vi "Sekvenca (SubVI).vi"(11 "Ulaz":dbl) -> (3 "Cluster 41":cluster{"Path":path, "Array":dbl[]})   [LabVIEW 2012]
panel:
  in  "Cluster 40":cluster{"Path":path, "Array":dbl[]}={"Path"=path "40.wav", "Array"=[1.0, 2.0]}
  in  "Cluster 39":cluster{"Path":path, "Array":dbl[]}={"Path"=path "39.wav", "Array"=[1.0, 2.0]}
  in  "Cluster 38":cluster{"Path":path, "Array":dbl[]}={"Path"=path "38.wav", "Array"=[1.0, 1.0, 2.0, 1.0]}
  in  "Cluster 37":cluster{"Path":path, "Array":dbl[]}={"Path"=path "37.wav", "Array"=[1.0, 1.0, 2.0, 1.0]}
  in  "Cluster 36":cluster{"Path":path, "Array":dbl[]}={"Path"=path "36.wav", "Array"=[2.0, 1.0]}
  in  "Cluster 35":cluster{"Path":path, "Array":dbl[]}={"Path"=path "35.wav", "Array"=[2.0, 1.0]}
  in  "Cluster 34":cluster{"Path":path, "Array":dbl[]}={"Path"=path "34.wav", "Array"=[4.0, 1.0]}
  in  "Cluster 33":cluster{"Path":path, "Array":dbl[]}={"Path"=path "33.wav", "Array"=[4.0]}
  in  "Cluster 32":cluster{"Path":path, "Array":dbl[]}={"Path"=path "32.wav", "Array"=[1.0]}
  in  "Cluster 31":cluster{"Path":path, "Array":dbl[]}={"Path"=path "31.wav", "Array"=[1.0]}
  in  "Cluster 30":cluster{"Path":path, "Array":dbl[]}={"Path"=path "30.wav", "Array"=[1.0]}
  in  "Cluster 29":cluster{"Path":path, "Array":dbl[]}={"Path"=path "29.wav", "Array"=[1.0]}
  in  "Cluster 28":cluster{"Path":path, "Array":dbl[]}={"Path"=path "28.wav", "Array"=[1.0, 1.0]}
  in  "Cluster 27":cluster{"Path":path, "Array":dbl[]}={"Path"=path "27.wav", "Array"=[1.0, 1.0]}
  in  "Cluster 26":cluster{"Path":path, "Array":dbl[]}={"Path"=path "26.wav", "Array"=[1.0, 1.0, 2.0]}
  in  "Cluster 25":cluster{"Path":path, "Array":dbl[]}={"Path"=path "25.wav", "Array"=[1.0, 1.0, 2.0]}
  in  "Cluster 24":cluster{"Path":path, "Array":dbl[]}={"Path"=path "24.wav", "Array"=[1.0, 1.0]}
  in  "Cluster 23":cluster{"Path":path, "Array":dbl[]}={"Path"=path "23.wav", "Array"=[1.0, 1.0]}
  in  "Cluster 22":cluster{"Path":path, "Array":dbl[]}={"Path"=path "22.wav", "Array"=[2.0, 3.0, 2.0]}
  in  "Cluster 21":cluster{"Path":path, "Array":dbl[]}={"Path"=path "21.wav", "Array"=[1.0, 1.0, 2.0]}
  in  "Cluster 20":cluster{"Path":path, "Array":dbl[]}={"Path"=path "20.wav", "Array"=[1.0, 1.0, 2.0, 1.0]}
  in  "Cluster 19":cluster{"Path":path, "Array":dbl[]}={"Path"=path "19.wav", "Array"=[1.0, 2.0, 1.0, 1.0]}
  in  "Cluster 18":cluster{"Path":path, "Array":dbl[]}={"Path"=path "18.wav", "Array"=[1.0, 2.0, 1.0]}
  in  "Cluster 17":cluster{"Path":path, "Array":dbl[]}={"Path"=path "17.wav", "Array"=[1.0, 2.0]}
  in  "Cluster 16":cluster{"Path":path, "Array":dbl[]}={"Path"=path "16.wav", "Array"=[1.0, 1.0, 1.0]}
  in  "Cluster 15":cluster{"Path":path, "Array":dbl[]}={"Path"=path "15.wav", "Array"=[1.0, 1.0]}
  in  "Cluster 14":cluster{"Path":path, "Array":dbl[]}={"Path"=path "14.wav", "Array"=[1.0, 1.0, 2.0]}
  in  "Cluster 13":cluster{"Path":path, "Array":dbl[]}={"Path"=path "13.wav", "Array"=[1.0, 1.0, 2.0]}
  in  "Cluster 12":cluster{"Path":path, "Array":dbl[]}={"Path"=path "12.wav", "Array"=[2.0, 1.0]}
  in  "Cluster 11":cluster{"Path":path, "Array":dbl[]}={"Path"=path "11.wav", "Array"=[1.0, 1.0, 2.0, 1.0, 1.0, 2.0]}
  in  "Cluster 10":cluster{"Path":path, "Array":dbl[]}={"Path"=path "10.wav", "Array"=[1.0, 1.0, 2.0, 1.0, 1.0, 2.0]}
  in  "Cluster 9":cluster{"Path":path, "Array":dbl[]}={"Path"=path "9.wav", "Array"=[1.0, 1.0, 2.0, 1.0, 1.0, 2.0]}
  in  "Cluster 8":cluster{"Path":path, "Array":dbl[]}={"Path"=path "8.wav", "Array"=[1.0, 1.0, 2.0, 1.0]}
  in  "Cluster 7":cluster{"Path":path, "Array":dbl[]}={"Path"=path "7.wav", "Array"=[2.0, 1.0]}
  in  "Cluster 6":cluster{"Path":path, "Array":dbl[]}={"Path"=path "6.wav", "Array"=[1.0, 2.0]}
  in  "Cluster 5":cluster{"Path":path, "Array":dbl[]}={"Path"=path "5.wav", "Array"=[1.0]}
  in  "Cluster 4":cluster{"Path":path, "Array":dbl[]}={"Path"=path "4.wav", "Array"=[1.0]}
  in  "Cluster 3":cluster{"Path":path, "Array":dbl[]}={"Path"=path "3.wav", "Array"=[1.0]}
  in  "Cluster 2":cluster{"Path":path, "Array":dbl[]}={"Path"=path "2.wav", "Array"=[1.0]}
  in  "Cluster 1":cluster{"Path":path, "Array":dbl[]}={"Path"=path "1.wav", "Array"=[1.0, 1.0, 2.0, 1.0]}
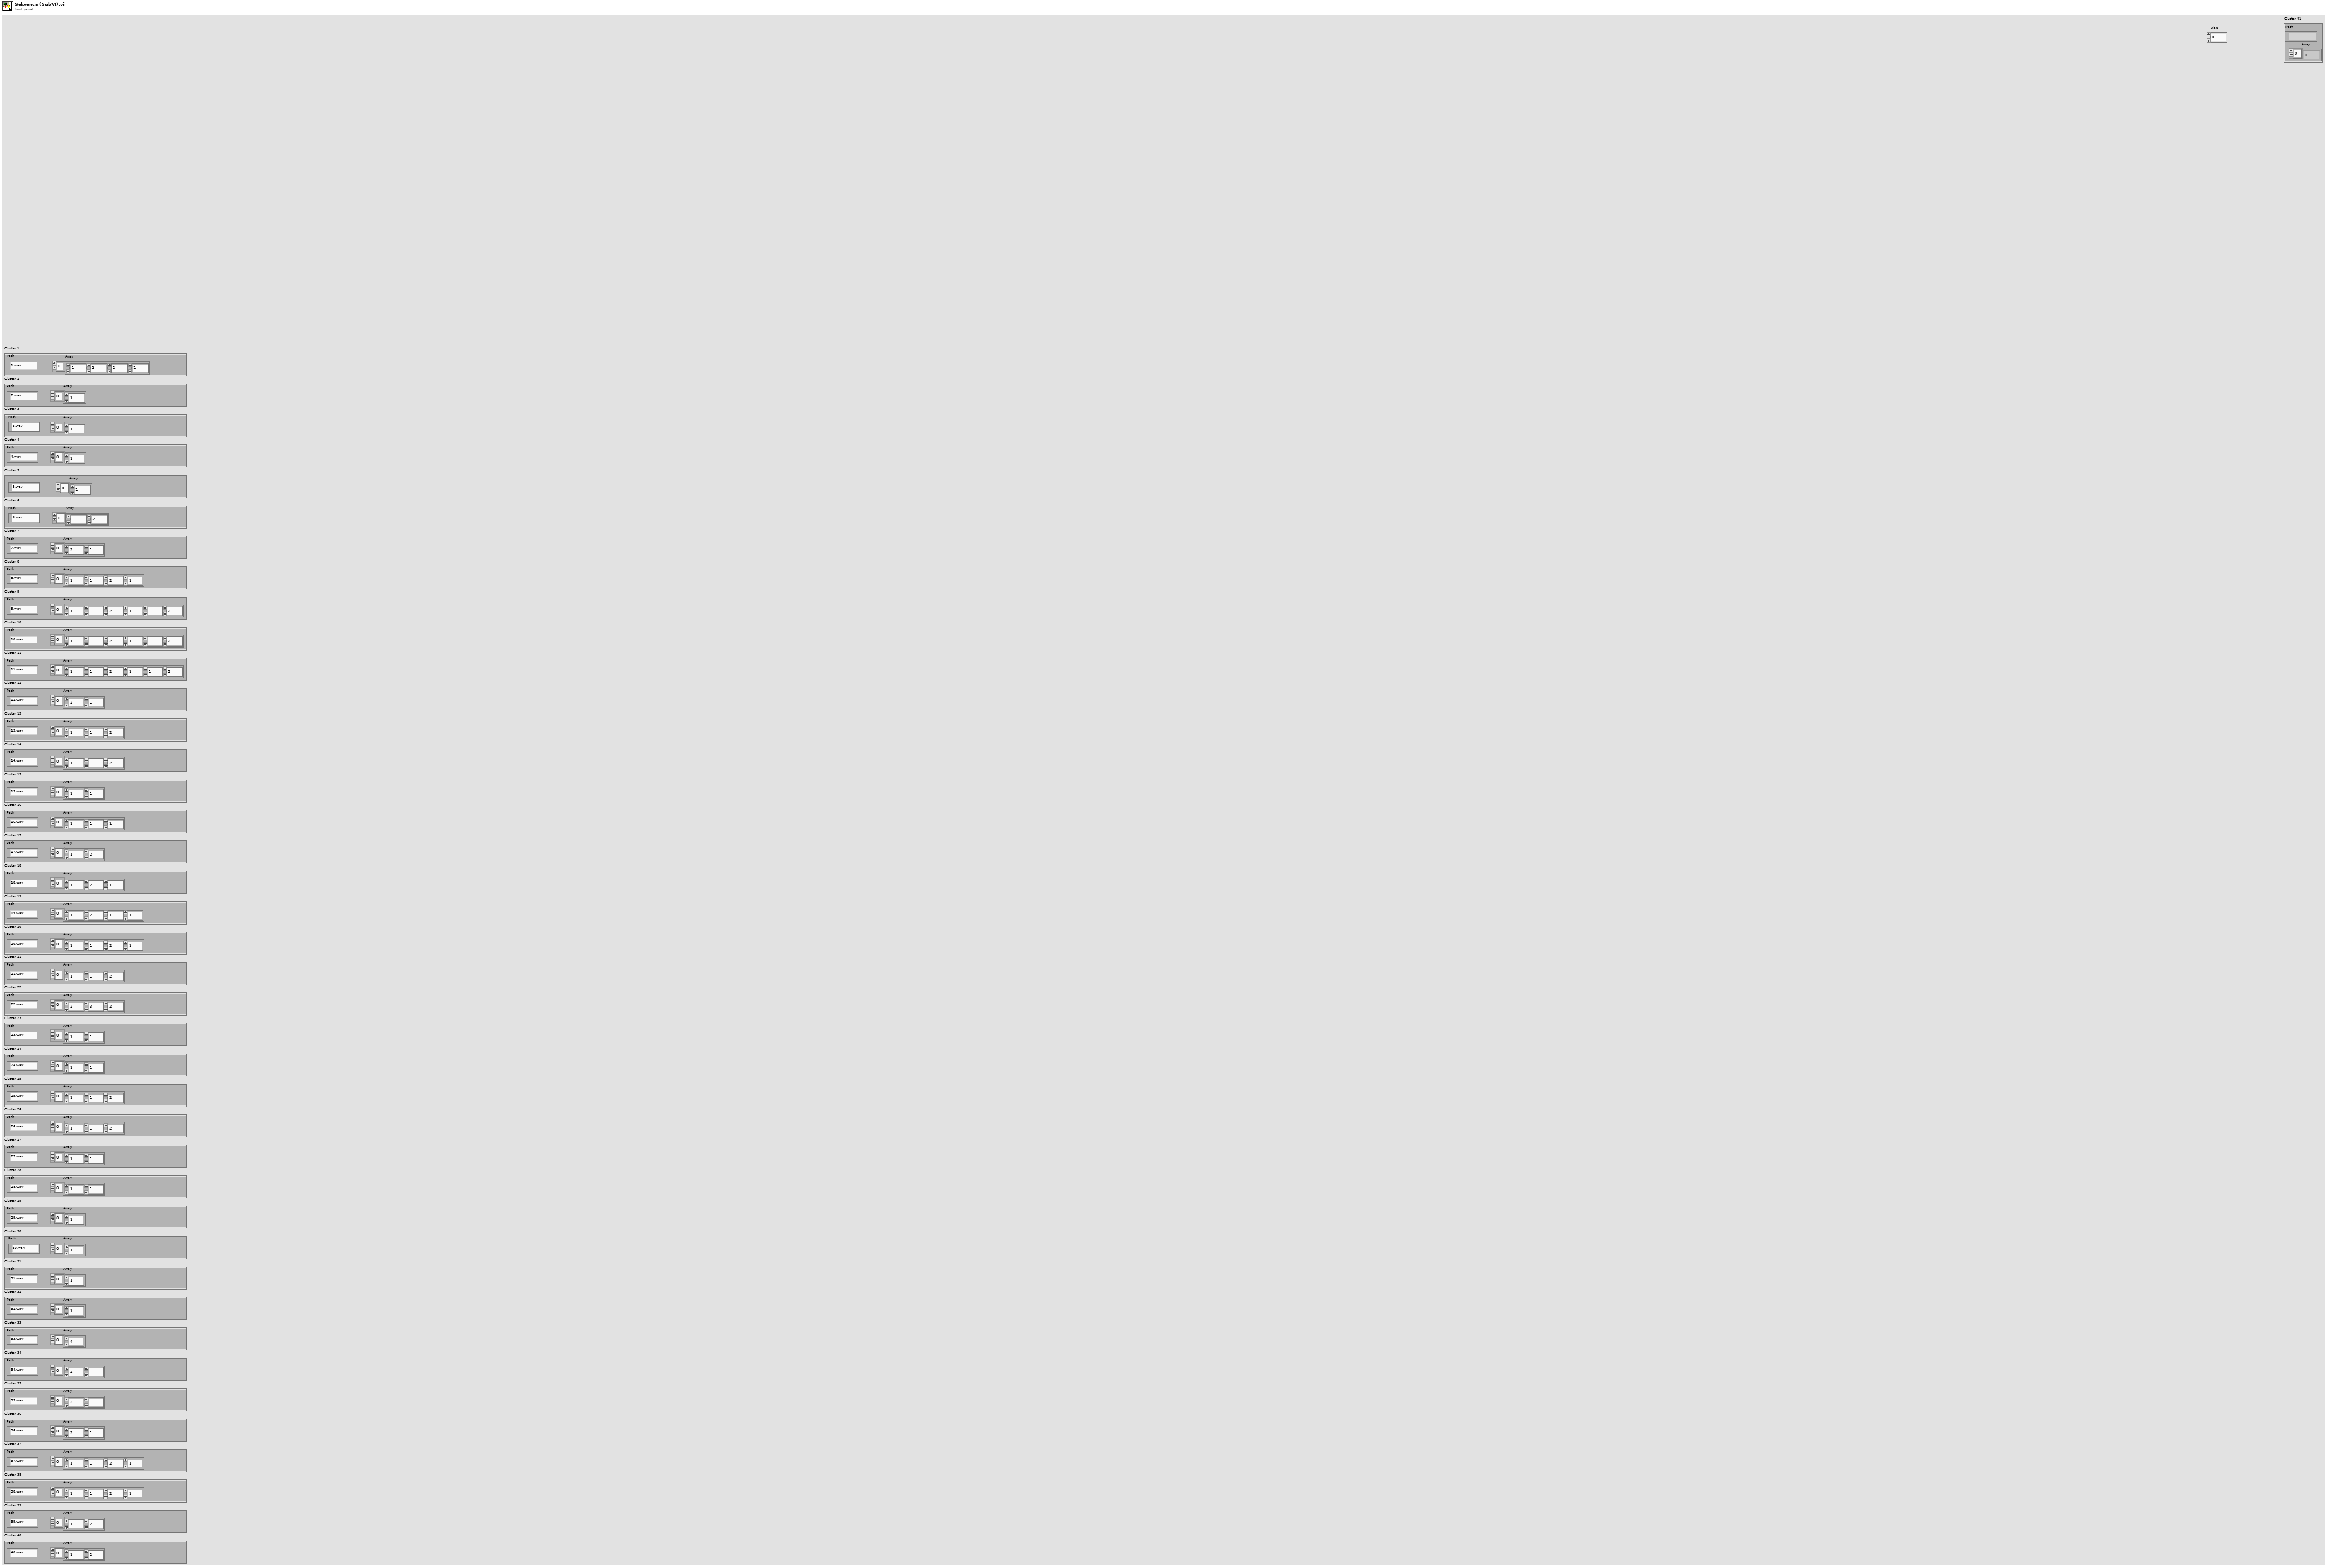
[diagram p1: front panel]
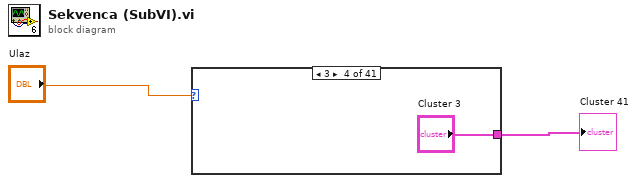
[diagram p0: block diagram]
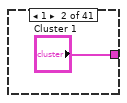
[diagram p3: hidden frame]
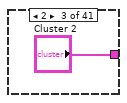
[diagram p4: hidden frame]
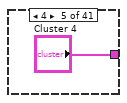
[diagram p5: hidden frame]
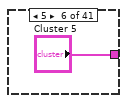
[diagram p6: hidden frame]
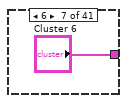
[diagram p7: hidden frame]
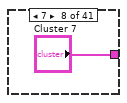
[diagram p8: hidden frame]
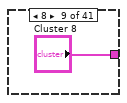
[diagram p9: hidden frame]
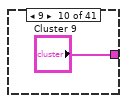
[diagram p10: hidden frame]
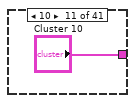
[diagram p11: hidden frame]
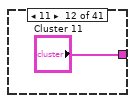
[diagram p12: hidden frame]
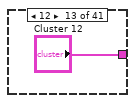
[diagram p13: hidden frame]
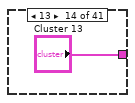
[diagram p14: hidden frame]
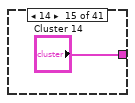
[diagram p15: hidden frame]
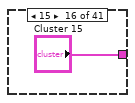
[diagram p16: hidden frame]
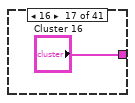
[diagram p17: hidden frame]
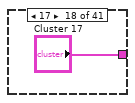
[diagram p18: hidden frame]
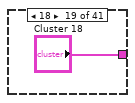
[diagram p19: hidden frame]
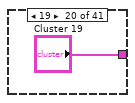
[diagram p20: hidden frame]
diagram:
  n1 = case shown="3" "Ulaz" {
    tunnel: [_ "Cluster 1" "Cluster 2" "Cluster 3" "Cluster 4" "Cluster 5" "Cluster 6" "Cluster 7" "Cluster 8" "Cluster 9" "Cluster 10" "Cluster 11" "Cluster 12" "Cluster 13" "Cluster 14" "Cluster 15" "Cluster 16" "Cluster 17" "Cluster 18" "Cluster 19" "Cluster 20" "Cluster 21" "Cluster 22" "Cluster 23" "Cluster 24" "Cluster 25" "Cluster 26" "Cluster 27" "Cluster 28" "Cluster 29" "Cluster 30" "Cluster 31" "Cluster 32" "Cluster 33" "Cluster 34" "Cluster 35" "Cluster 36" "Cluster 37" "Cluster 38" "Cluster 39" "Cluster 40"] -> w1
    frame 0, Default {
    }
    frame 1 {
    }
    frame 2 {
    }
    frame 3 {
    }
    frame 4 {
    }
    frame 5 {
    }
    frame 6 {
    }
    frame 7 {
    }
    frame 8 {
    }
    frame 9 {
    }
    frame 10 {
    }
    frame 11 {
    }
    frame 12 {
    }
    frame 13 {
    }
    frame 14 {
    }
    frame 15 {
    }
    frame 16 {
    }
    frame 17 {
    }
    frame 18 {
    }
    frame 19 {
    }
    frame 20 {
    }
    frame 21 {
    }
    frame 22 {
    }
    frame 23 {
    }
    frame 24 {
    }
    frame 25 {
    }
    frame 26 {
    }
    frame 27 {
    }
    frame 28 {
    }
    frame 29 {
    }
    frame 30 {
    }
    frame 31 {
    }
    frame 32 {
    }
    frame 33 {
    }
    frame 34 {
    }
    frame 35 {
    }
    frame 36 {
    }
    frame 37 {
    }
    frame 38 {
    }
    frame 39 {
    }
    frame 40 {
    }
  }
  "Cluster 41" <- w1
